vi "Control ITC Sweep -- initialize aggregate state.vi"(6 "time step":i32, 8 "error in":errorcluster, 10 "length":i32, 11 "more state -- aggregate in":T1={"time(min)"=array[7200 elements], "T (ITC )"=array[7200 elements], "T (ITC, set)"=array[7200 elements], "T (LTC)"=array[7200 elements], "heater"=array[7200 elements], "gas"=array[7200 elements], "T (ITC)  - T (ITC, set)"=array[7200 elements], "T (LTC)  - T (ITC, set)"=array[7200 elements], "heater slope"=array[7200 elements], "LTC slope"=array[7200 elements], "hetaer running average"=array[7200 elements], "T (LTC) running average"=array[7200 elements]}) -> (0 "error out":errorcluster, 3 "more state -- aggregate out":T1)   [LabVIEW 2010]
uses:
  collect.ctl
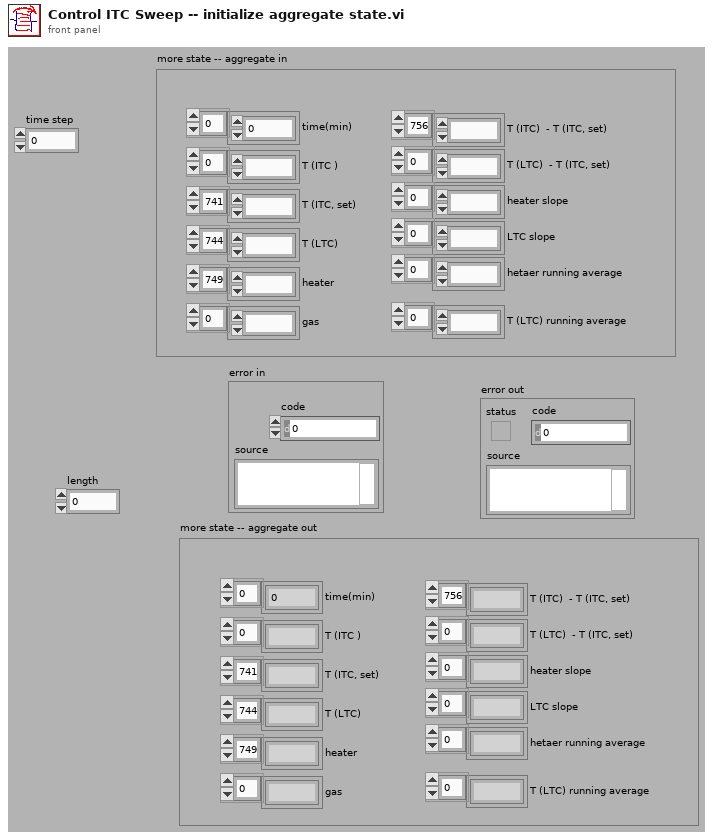
[diagram p1: front panel]
types:
  T1 = typedef "collect.ctl" = cluster{"time(min)":dbl[], "T (ITC )":dbl[], "T (ITC, set)":dbl[], "T (LTC)":dbl[], "heater":dbl[], "gas":dbl[], "T (ITC)  - T (ITC, set)":dbl[], "T (LTC)  - T (ITC, set)":dbl[], "heater slope":dbl[], "LTC slope":dbl[], "hetaer running average":dbl[], "T (LTC) running average":dbl[]}
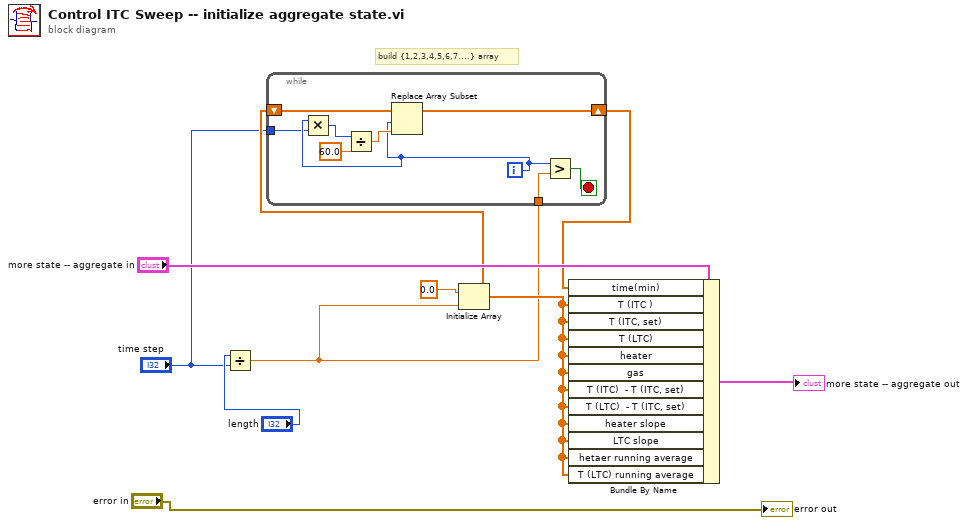
[diagram p0: block diagram]
diagram:
  # "build {1,2,3,4,5,6,7....} array"
  n1 = Divide(x="length", y="time step") -> (x/y=w2:dbl)
  n2 = Initialize Array(0.0 ("element"), w2) -> (w5:dbl[])
  n3 = while {
    tunnel: w2 -> [w17]
    shift-right: [w13] -> w4
    shift-left: w5 -> [w16]
    tunnel: "time step" -> [w11]
    i -> [w12]
    stop <- w18 stop-if-true
    n4 = Multiply(x=w12, y=w11) -> (x*y=w10:i32)
    n5 = Divide(x=w10, y=60.0) -> (x/y=w15:dbl)
    n6 = Replace Array Subset(array=w16, new element=w15, index=w12) -> (w13:dbl[])
    n7 = Greater?(x=w12, y=w17) -> (0:w18:bool)
  }
  n8 = Bundle By Name(cluster="more state -- aggregate in", "time(min)"=w4, "T (ITC )"=w5, "T (ITC, set)"=w5, "T (LTC)"=w5, "heater"=w5, "gas"=w5, "T (ITC)  - T (ITC, set)"=w5, "T (LTC)  - T (ITC, set)"=w5, "heater slope"=w5, "LTC slope"=w5, "hetaer running average"=w5, "T (LTC) running average"=w5) -> (→"more state -- aggregate out":T1)
  "error out" <- "error in"
